vi "Wait For Bytes.vi"(7 "Timeout (100 ms)":u32=100, 8 "Error In":errorcluster, 10 "Num Bytes":u32, 11 "LINX Device Config":T1) -> (0 "Error Out":errorcluster, 1 "Timeout":bool, 2 "Num Bytes":u32, 3 "LINX Device Config":T1)   [LabVIEW 2011, in "LVH-LINX.lvlib"]
doc: "Wait until the specified number of bytes are abailable at the serial port or a timeout occurs."
uses:
  LVH-LINX.lvlib
  Type Defs/LINX Device Config.ctl
  Type Defs/Interface.ctl
  Type Defs/TCP Config.ctl
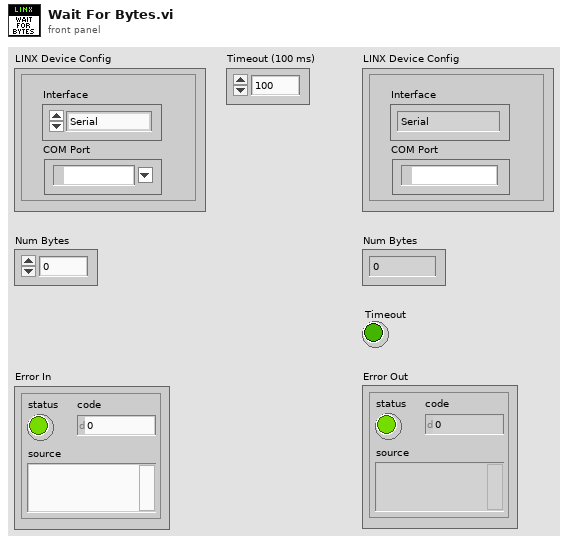
[diagram p1: front panel]
types:
  T1 = typedef "LVH-LINX.lvlib/LINX Device Config.ctl" = cluster{"Interface":T2, "COM Port":refnum<visa-resource-name>, "Packet Number":u16, "TCP Configuration":T3}
  T2 = typedef "LVH-LINX.lvlib/Interface.ctl" = enum16{"Serial", "TCP"}
  T3 = typedef "LVH-LINX.lvlib/TCP Config.ctl" = cluster{"IP Address":string, "Port":dbl}
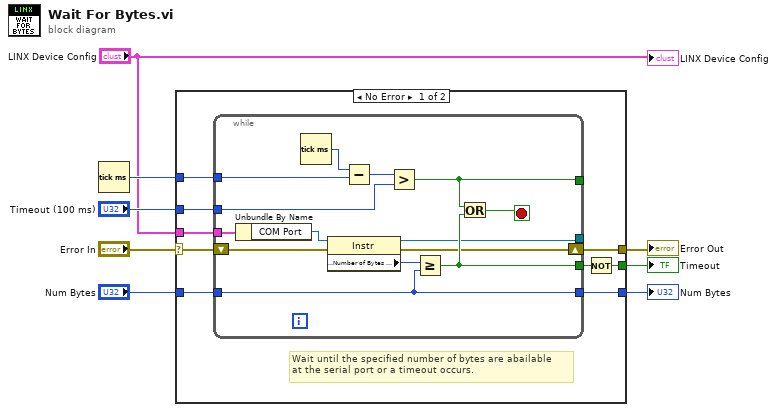
[diagram p0: block diagram]
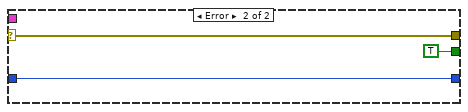
[diagram p2: hidden frame]
diagram:
  n1 = Tick Count (ms)() -> (millisecond timer value=w6:u32)
  n2 = case shown="No Error" "Error In" {
    selector: "Error In" -> [w11 w34]
    tunnel: [w17 w34] -> w8
    tunnel: "LINX Device Config" -> [w16 _]
    tunnel: "Timeout (100 ms)" -> [w15 _]
    tunnel: w6 -> [w14 _]
    tunnel: [w9 TRUE] -> w1
    tunnel: "Num Bytes" -> [w13 w33]
    tunnel: [w12 w33] -> w4
    frame No Error {
      # "Wait until the specified number of bytes are abailable\nat the serial port or a timeout occurs."
      n3 = while {
        tunnel: w14 -> [w30]
        tunnel: w15 -> [w28]
        tunnel: w16 -> [w19]
        shift-right: [w22] -> w17
        shift-left: w11 -> [w27]
        tunnel: [w24] -> w10
        tunnel: [w25] -> _
        tunnel: [w21] -> _
        tunnel: w13 -> [w20]
        tunnel: [w20] -> w12
        stop <- w23 stop-if-true
        n4 = Unbundle By Name(w19) -> ("COM Port"=w18:refnum<visa-resource-name>)
        n5 = Tick Count (ms)() -> (millisecond timer value=w31:u32)
        n6 = property class="Instr"(reference=w18, error in=w27) -> (reference out=w21:refnum<visa-resource-name>, error out=w22:errorcluster, "Serial Settings:Number of Bytes at Serial Port"=w26:u32)
        n7 = Subtract(x=w31, y=w30) -> (x-y=w29:u32)
        n8 = Greater?(x=w29, y=w28) -> (0:w25:bool)
        n9 = Greater Or Equal?(x=w26, y=w20) -> (x >= y?=w24:bool)
        n10 = Or(x=w25, y=w24) -> (x .or. y?=w23:bool)
      }
      n11 = Not(x=w10) -> (.not. x?=w9:bool)
    }
    frame Error {
    }
  }
  "Error Out" <- w8
  "Timeout" <- w1
  "Num Bytes" <- w4
  "LINX Device Config" <- "LINX Device Config"
